vi "UA_Node Quene.vi"(8 "error in (no error)":errorcluster caption="错误输入（无错误）", 9 "node in":T1, 11 "OP Action":T2) -> (0 "error out":errorcluster caption="错误输出", 1 "node out":T1, 3 "Qune Lenth":i32)   [LabVIEW 2013]
uses:
  UA_Node.ctl
  UA_OP Action.ctl
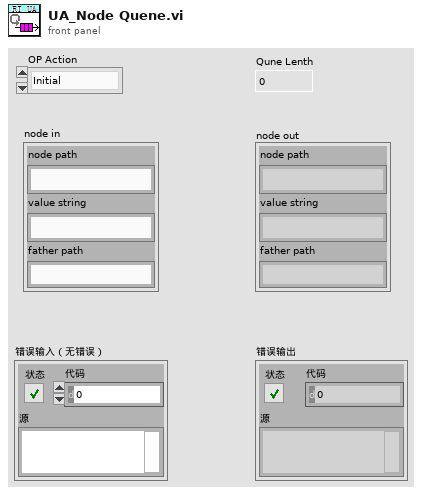
[diagram p1: front panel]
types:
  T1 = typedef "UA_Node.ctl" = cluster{"node path":string, "value string":string, "father path":string}
  T2 = typedef "UA_OP Action.ctl" = enum16{"Initial", "Add node", "Get node", "Get length", "View node"}
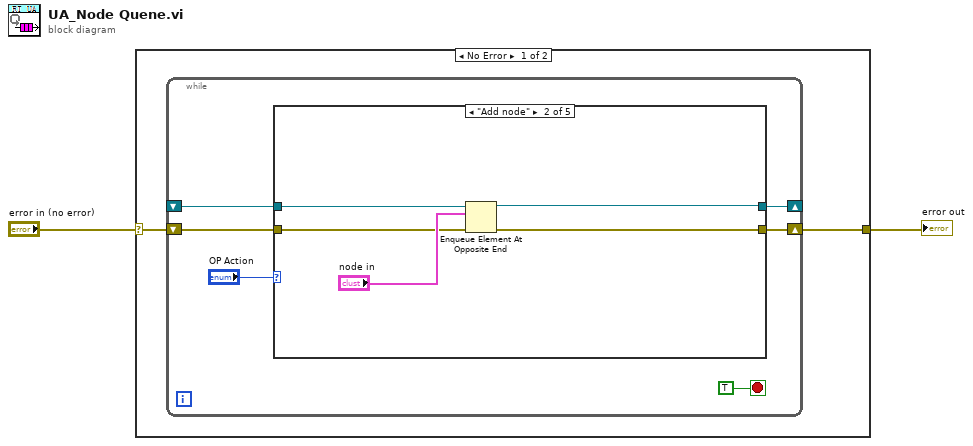
[diagram p0: block diagram]
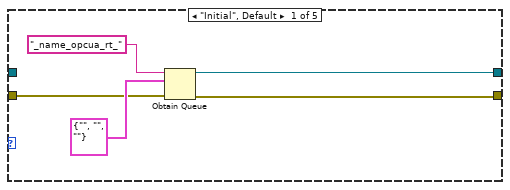
[diagram p2: hidden frame]
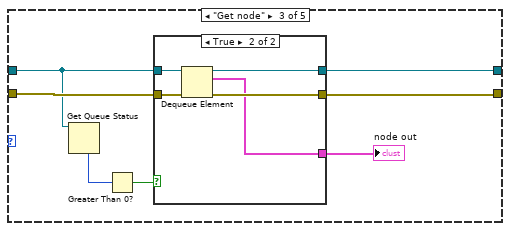
[diagram p3: hidden frame]
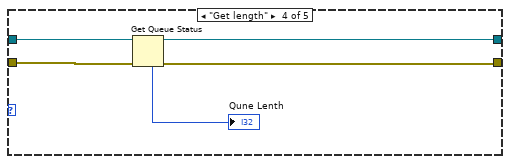
[diagram p5: hidden frame]
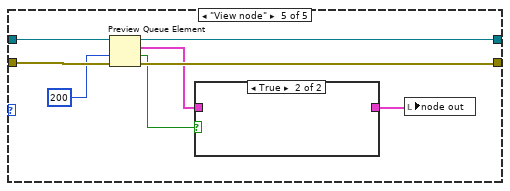
[diagram p6: hidden frame]
diagram:
  n1 = case shown="No Error" "error in (no error)" {
    selector: "error in (no error)" -> [w4 w49]
    tunnel: [w3 w49] -> w1
    frame No Error {
      n2 = while {
        shift-right: [w10] -> _
        shift-left: _ -> [w8]
        shift-right: [w7] -> w3
        shift-left: w4 -> [w6]
        stop <- TRUE stop-if-true
        n3 = case shown="\"Add node\"" "OP Action" {
          tunnel: [w15 w19 w26 w36 w45] -> w10
          tunnel: w8 -> [_ w20 w24 w39 w47]
          tunnel: [w13 w17 w25 w37 w44] -> w7
          tunnel: w6 -> [w12 w16 w27 w38 w46]
          frame "Initial", Default {
            n4 = Obtain Queue(name (unnamed)="_name_opcua_rt_" ("名称（未命名）"), element data type=T1 {"node path"="", "value string"="", "father path"=""} ("node"), error in (no error)=w12) -> (queue out=w15:refnum<queue>, error out=w13:errorcluster)  [unwired: 2 in, 1 out]
          }
          frame "Add node" {
            n5 = Enqueue Element At Opposite End(queue=w20, element="node in", error in (no error)=w16) -> (queue out=w19:refnum<queue>, error out=w17:errorcluster)  [unwired: 1 in, 1 out]
          }
          frame "Get node" {
            n6 = Get Queue Status(queue=w24) -> (# elements in queue=w23:i32)  [unwired: 2 in, 7 out]
            n7 = Greater Than 0?(x=w23) -> (x > 0?=w22:bool)
            n8 = case shown="True" w22 {
              tunnel: w27 -> [w28 w34]
              tunnel: [w29 w33] -> w26
              tunnel: [w28 w32] -> w25
              tunnel: w24 -> [w29 w31]
              tunnel: [_ w30] -> w21
              frame False {
              }
              frame True {
                n9 = Dequeue Element(queue=w31, error in (no error)=w34) -> (queue out=w33:refnum<queue>, element=w30:T1, error out=w32:errorcluster)  [unwired: 1 in, 1 out]
              }
            }
            "node out" <- w21
          }
          frame "Get length" {
            n10 = Get Queue Status(queue=w39, error in (no error)=w38) -> (queue out=w36:refnum<queue>, error out=w37:errorcluster, # elements in queue=→"Qune Lenth":i32)  [unwired: 1 in, 5 out]
          }
          frame "View node" {
            n11 = Preview Queue Element(queue=w47, timeout in ms (-1)=200 ("超时毫秒(-1)"), error in (no error)=w46) -> (queue out=w45:refnum<queue>, element=w43:T1, timed out?=w41:bool, error out=w44:errorcluster)
            n12 = case shown="True" w41 {
              tunnel: w43 -> [w48 _]
              tunnel: [w48 _] -> w40
              frame False {
              }
              frame True {
              }
            }
            n13 = local write "node out"(w40) -> ()
          }
        }
      }
    }
    frame Error {
    }
  }
  "error out" <- w1
